vi "Write Base Actor DVR.vi"(10 "Base Actor DVR":refnum<data-value>, 11 "Base Actor in":refnum<class "Base Actor.lvclass">) -> (3 "Base Actor out":refnum<class "Base Actor.lvclass">)   [LabVIEW 2020, in "jettl.lvlib" / "Base jettl Actor.lvlib" / "Base Actor.lvlib" / "Base Actor.lvclass"]
uses:
  Base Actor.lvclass
  Base Actor.lvclass/Base Actor.ctl
  Msg/Msg.lvclass
  Unified Actor Lifetime.ctl
  jettl.lvlib
  Base Actor.ctl
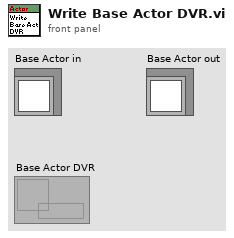
[diagram p1: front panel]
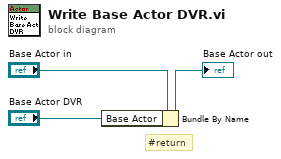
[diagram p0: block diagram]
diagram:
  # "#return"
  n1 = Bundle By Name(cluster="Base Actor in", "Base Actor"="Base Actor DVR") -> (→"Base Actor out":refnum<class "Base Actor.lvclass">)
